vi "Парал Рег 4.vi"(0 "C":bool, 2 "Reset":bool, 3 "D":T1) -> (1 "Q":T2)   [LabVIEW 2017]
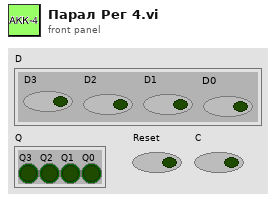
[diagram p1: front panel]
types:
  T1 = cluster{"D3":bool, "D2":bool, "D1":bool, "D0":bool}
  T2 = cluster{"Q3":bool, "Q2":bool, "Q1":bool, "Q0":bool}
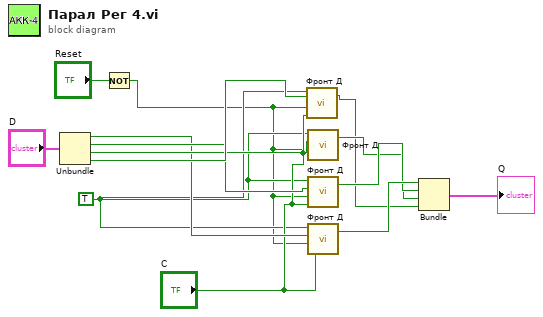
[diagram p0: block diagram]
diagram:
  w7 = TRUE
  n1 = Unbundle("D") -> ("D3"=w10:bool, "D2"=w11:bool, "D1"=w12:bool, "D0"=w13:bool)
  n2 = Not(x="Reset") -> (.not. x?=w6:bool)
  n3 = call "Фронт Д.vi"("C"="C", "S"=w6, "D"=w13, "R"=w7) -> ("Q"=w2:bool)  [unwired: 1 out]
  n4 = call "Фронт Д.vi"("C"="C", "S"=w6, "D"=w12, "R"=w7) -> ("Q"=w3:bool)  [unwired: 1 out]
  n5 = call "Фронт Д.vi"("C"="C", "S"=w6, "D"=w11, "R"=w7) -> ("Q"=w4:bool)  [unwired: 1 out]
  n6 = call "Фронт Д.vi"("C"="C", "S"=w6, "D"=w10, "R"=w7) -> ("Q"=w5:bool)  [unwired: 1 out]
  n7 = Bundle("Q"=w5, "Q"=w4, "Q"=w3, "Q"=w2) -> (→"Q":cluster{"Q":bool, "Q":bool, "Q":bool, "Q":bool})  [unwired: 1 in]
